vi "TeleOp Shooter.vi"() -> ()   [LabVIEW 2020]
uses:
  <vilib>/Rock Robotics/WPI/Utilities/WPI_GetSetVariantRefNum.vi
  7fd68e31-625e-414b-937c-b349f460b20b.vi
panel:
  in  "Numeric":dbl=0.4
  out "Proximity 1":u16
  out "Proximity 2":u16
  in  "Proximity comparison":u16=100
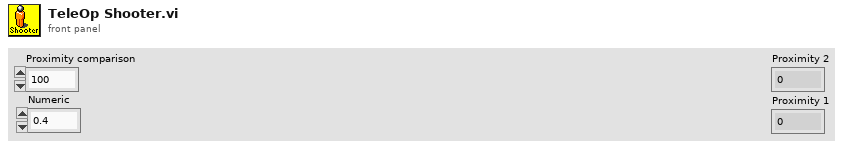
[diagram p1: front panel]
types:
  T1 = typedef "WPI_JoystickDevRef.ctl" = cluster{"Device":T2}
  T2 = typedef "WPI_JoystickDeviceEnum.ctl" = enum16{"USB 0", "USB 1", "USB 2", "USB 3", "USB 4", "USB 5"}
  T3 = typedef "Color Sensor V3 DevRef.ctl" = cluster{"I2CDevRef":T4}
  T4 = typedef "WPI_I2CDevRef.ctl" = cluster{"DevStatus":errorcluster, "Device Address":u8, "Handle":i32, "I2C Bus":T5}
  T5 = typedef "i2c_bus.ctl" = enum16{"I2C On-Board", "I2C MXP", "Invalid"}
  T6 = typedef "WPI_MotorControlDeviceRef.ctl" = cluster{"DeviceStatus":errorcluster, "Type":T7, "PWM":cluster{"PWM Channel":T8, "DeadBand":T9}, "CAN":cluster{"Device Number":u8, "SetOutput VI Ref":variant, "GetOutput VI Ref":variant, "Enable VI Ref":variant, "Disable VI Ref":variant, "Data":variant}, "Invert":bool, "DIO PWM":cluster{"PWM \"Enable\" Channel":T8, "DIOChannel":T10, "PWM Rate":dbl}}
  T7 = typedef "WPI_MotorControlType.ctl" = enum16{"PWM", "CAN", "DIO PWM"}
  T8 = typedef "FPGA_DIOPWMChannel.ctl" = enum8{"PWM 0", "PWM 1", "PWM 2", "PWM 3", "PWM 4", "PWM 5", "PWM 6", "PWM 7", "PWM 8", "PWM 9", "PWM MXP 0", "PWM MXP 1", "PWM MXP 2", "PWM MXP 3", "PWM MXP 4", "PWM MXP 5", "PWM MXP 6", "PWM MXP 7", "PWM MXP 8", "PWM MXP 9", "Invalid"}
  T9 = typedef "WPI_PWMDeadband.ctl" = cluster{"Name":string, "maxPositivePwm":i32, "minPositivePwm":i32, "centerPwm":i32, "maxNegativePwm":i32, "minNegativePwm":i32, "angularRange":u16}
  T10 = typedef "FPGA_DIOChannel.ctl" = enum8{"DIO 0", "DIO 1", "DIO 2", "DIO 3", "DIO 4", "DIO 5", "DIO 6", "DIO 7", "DIO 8", "DIO 9", "DIO MXP 0", "DIO MXP 1", "DIO MXP 2", "DIO MXP 3", "DIO MXP 4", "DIO MXP 5", "DIO MXP 6", "DIO MXP 7", "DIO MXP 8", "DIO MXP 9", "DIO MXP 10", "DIO MXP 11", "DIO MXP 12", "DIO MXP 13", "DIO MXP 14", "DIO MXP 15", "SPI Port CS1", "SPI Port CS2", "SPI Port CS3", "SPI Port MISO", "SPI Port MOSI", "Invalid"}
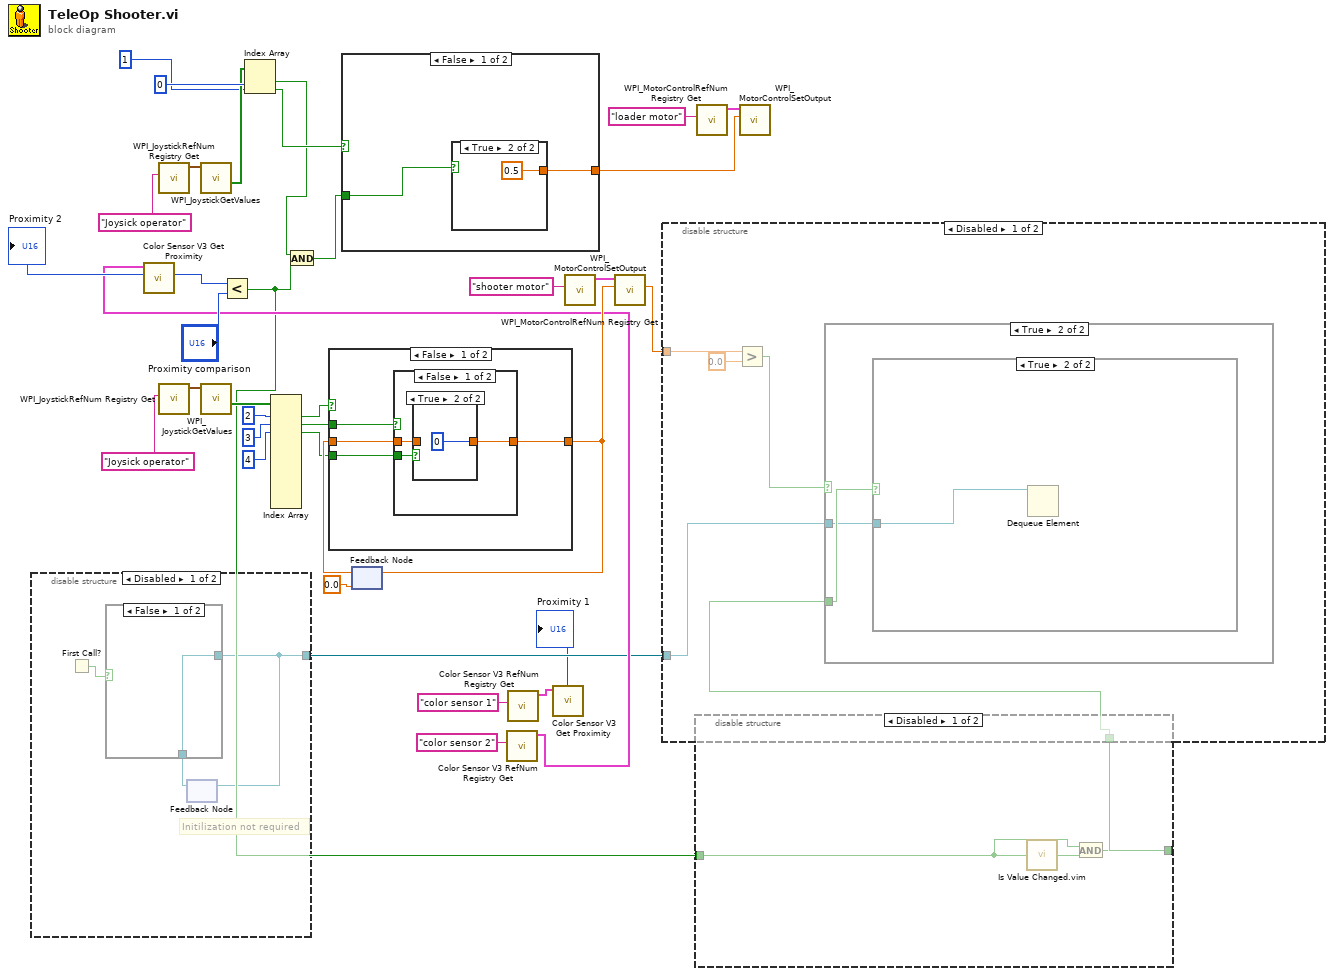
[diagram p0: block diagram]
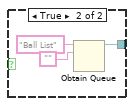
[diagram p3: hidden frame]
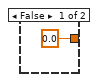
[diagram p8: hidden frame]
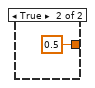
[diagram p9: hidden frame]
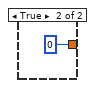
[diagram p11: hidden frame]
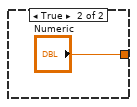
[diagram p12: hidden frame]
diagram:
  n1 = disable-structure shown="Disabled" {
    disable-tunnel: [w38 _] -> w3
    frame Disabled {
      # "Initilization not required"
      n2 = First Call?() -> (First Call?: T/F=w39:bool)
      n3 = feedback #1() -> (w37:refnum<queue>)  [unwired: 1 in]
      n4 = case shown="False" w39 {
        tunnel: [w40 w41] -> w38
        tunnel: w37 -> [w40 _]
        frame False {
        }
        frame True {
          n5 = Obtain Queue(name (unnamed)="Ball List", element data type="") -> (queue out=w41:refnum<queue>)  [unwired: 3 in, 2 out]
        }
      }
      n6 = feedback-in #1(w38) -> ()
    }
    frame Enabled {
    }
  }
  n7 = call <vilib>:"WPI_JoystickRefNum Registry Get.vi"("refnum name"="Joysick operator") -> ("JoystickDevRef"=w33:T1)  [unwired: 9 in, 1 out]
  n8 = call <vilib>:"WPI_JoystickRefNum Registry Get.vi"("refnum name"="Joysick operator") -> ("JoystickDevRef"=w27:T1)  [unwired: 9 in, 1 out]
  n9 = call <vilib>:"WPI_JoystickGetValues.vi"("JoystickDevRef"=w33) -> ("Buttons"=w34:bool[])  [unwired: 6 in, 4 out]
  n10 = call <vilib>:"WPI_JoystickGetValues.vi"("JoystickDevRef"=w27) -> ("Buttons"=w21:bool[])  [unwired: 6 in, 4 out]
  n11 = Index Array(array=w34, index #1=0 ("index"), index #2=1 ("index")) -> (element #1=w7:bool, element #2=w12:bool)
  n12 = Index Array(array=w21, index #1=2 ("index"), index #2=3 ("index"), index #3=4 ("index")) -> (element #1=w18:bool, element #2=w17:bool, element #3=w16:bool)  [unwired: 9 in, 9 out]
  n13 = feedback #2(0.0) -> (w23:dbl)
  n14 = case shown="False" w18 {
    tunnel: [w47 "Numeric"] -> w24
    tunnel: w23 -> [w46 _]
    tunnel: w17 -> [w45 _]
    tunnel: w16 -> [w44 _]
    frame False {
      n15 = case shown="False" w45 {
        tunnel: [w50 0] -> w47
        tunnel: w46 -> [w49 _]
        tunnel: w44 -> [w48 _]
        frame False {
          n16 = case shown="True" w48 {
            tunnel: [w51 0] -> w50
            tunnel: w49 -> [w51 _]
            frame False {
            }
            frame True {
            }
          }
        }
        frame True {
        }
      }
    }
    frame True {
    }
  }
  n17 = feedback-in #2(w24) -> ()
  n18 = call <vilib>:"Color Sensor V3 RefNum Registry Get.vi"("refnum name"="color sensor 2") -> ("ColorSensorDevRef"=w6:T3)  [unwired: 9 in, 1 out]
  n19 = call <vilib>:"Color Sensor V3 Get Proximity.vi"("ColorSensorDevRef"=w6) -> ("Proximity"=w10:u16)  [unwired: 8 in, 2 out]
  "Proximity 2" <- w10
  n20 = Less?(x=w10, y="Proximity comparison") -> (x < y?=w4:bool)
  n21 = And(x=w7, y=w4) -> (x .and. y?=w8:bool)
  n22 = case shown="False" w12 {
    tunnel: [w56 0.5] -> w36
    tunnel: w8 -> [w55 _]
    frame False {
      n23 = case shown="True" w55 {
        tunnel: [0.0 0.5] -> w56
        frame False {
        }
        frame True {
        }
      }
    }
    frame True {
    }
  }
  n24 = call <vilib>:"Color Sensor V3 RefNum Registry Get.vi"("refnum name"="color sensor 1") -> ("ColorSensorDevRef"=w2:T3)  [unwired: 9 in, 1 out]
  n25 = call <vilib>:"Color Sensor V3 Get Proximity.vi"("ColorSensorDevRef"=w2) -> ("Proximity"=→"Proximity 1":u16)  [unwired: 8 in, 2 out]
  n26 = call <vilib>:"WPI_MotorControlRefNum Registry Get.vi"("refnum name"="shooter motor") -> ("MotorControlDevRef"=w25:T6)  [unwired: 9 in, 1 out]
  n27 = call <vilib>:"WPI_MotorControlSetOutput.vi"("Output"=w24, "MotorControlDevRef"=w25) -> ("Motor Output"=w15:dbl)  [unwired: 7 in, 2 out]
  n28 = disable-structure shown="Disabled" {
    disable-tunnel: [w61 _] -> w5
    disable-tunnel: w4 -> [w60 _]
    frame Disabled {
      n29 = call "Is Value Changed.vim"("value"=w60) -> ("changed or first call?"=w62:bool)
      n30 = And(x=w60, y=w62) -> (x .and. y?=w61:bool)
    }
    frame Enabled {
    }
  }
  n31 = disable-structure shown="Disabled" {
    disable-tunnel: w15 -> [w67 _]
    disable-tunnel: w5 -> [w64 _]
    disable-tunnel: w3 -> [w63 _]
    frame Disabled {
      n32 = Greater?(x=w67, y=0.0) -> (0:w65:bool)
      n33 = case shown="True" w65 {
        tunnel: w64 -> [_ w69]
        tunnel: w63 -> [_ w68]
        frame False {
        }
        frame True {
          n34 = case shown="True" w69 {
            tunnel: w68 -> [_ w70]
            frame False {
            }
            frame True {
              n35 = Dequeue Element(queue=w70) -> ()  [unwired: 2 in, 4 out]
            }
          }
        }
      }
    }
    frame Enabled {
    }
  }
  n36 = call <vilib>:"WPI_MotorControlRefNum Registry Get.vi"("refnum name"="loader motor") -> ("MotorControlDevRef"=w31:T6)  [unwired: 9 in, 1 out]
  n37 = call <vilib>:"WPI_MotorControlSetOutput.vi"("Output"=w36, "MotorControlDevRef"=w31) -> ()  [unwired: 7 in, 3 out]
